vi "Listener_Paralelo.vi"() -> ()   [LabVIEW 2019]
panel:
  out "error out":errorcluster
  out "Novo ID":refnum<k5>
  in  "[ESC]":bool
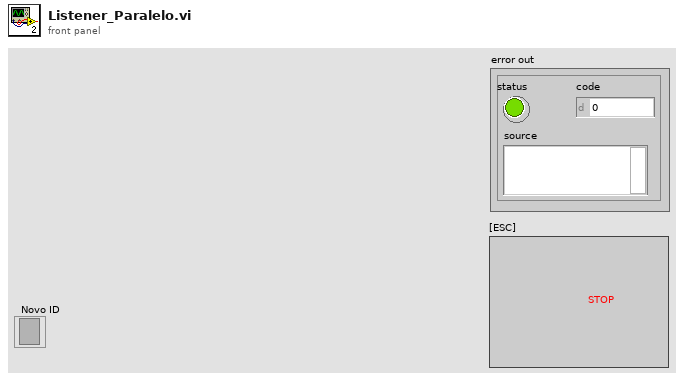
[diagram p1: front panel]
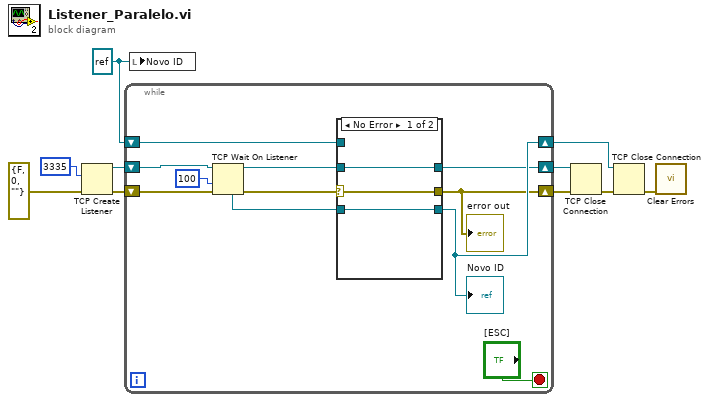
[diagram p0: block diagram]
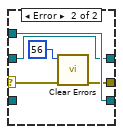
[diagram p2: hidden frame]
diagram:
  w6 = refnum<k5> refnum ("listener ID")
  n1 = TCP Create Listener(8:errorcluster {"status"=FALSE, "code"=0, "source"=""} ("error in (no error)"), 10:u16 3335 ("port")) -> (0:w8:errorcluster, 3:w7:refnum<k5>)  [unwired: 3 in, 1 out]
  n2 = while {
    shift-right: [w11] -> w5
    shift-left: w8 -> [w19]
    shift-right: [w13] -> w4
    shift-left: w7 -> [w18]
    shift-right: [w14] -> w3
    shift-left: w6 -> [w15]
    stop <- "[ESC]" stop-if-true
    n3 = TCP Wait On Listener(8:w19, 9:100 ("timeout ms (wait forever: -1)"), 11:w18) -> (0:w17:errorcluster, 3:w12:refnum<k5>, 4:w16:refnum<k5>)  [unwired: 3 out]
    n4 = case shown="No Error" w17 {
      selector: w17 -> [w23 w27]
      tunnel: w16 -> [w22 _]
      tunnel: w15 -> [_ w29]
      tunnel: [w22 w29] -> w14
      tunnel: w12 -> [w24 w28]
      tunnel: [w24 w28] -> w13
      tunnel: [w23 w25] -> w11
      frame No Error {
      }
      frame Error {
        n5 = call <vilib>:"Clear Errors.vi"("error in (no error)"=w27, "specific error code to clear (0: all)"=56) -> ("error out"=w25:errorcluster)  [unwired: 4 in, 1 out]
      }
    }
    "Novo ID" <- w14
    "error out" <- w11
  }
  n6 = local write "Novo ID"(w6) -> ()
  n7 = TCP Close Connection(connection ID=w4, error in (no error)=w5) -> (error out=w2:errorcluster)  [unwired: 1 in, 1 out]
  n8 = TCP Close Connection(connection ID=w3, error in (no error)=w2) -> (error out=w1:errorcluster)  [unwired: 1 in, 1 out]
  n9 = call <vilib>:"Clear Errors.vi"("error in (no error)"=w1) -> ()  [unwired: 5 in, 2 out]
